vi "readCSV.vi"() -> ()   [LabVIEW 2020]
uses:
  <vilib>/Utility/file.llb/Read Delimited Spreadsheet (string).vi
panel:
  in  "Numeric 2":dbl
  out "Numeric":dbl
  out "String 3":string
  out "String 2":string
  out "Array":T1(array[cluster])
  in  "String":string
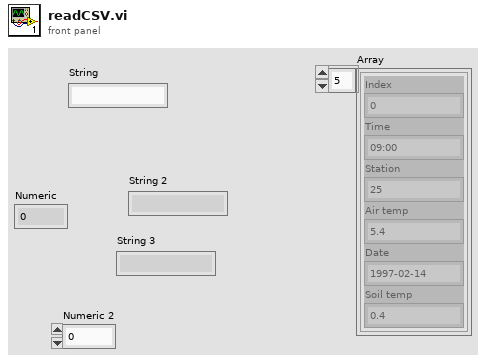
[diagram p1: front panel]
types:
  T1 = cluster{"Index":string, "Time":string, "Station":string, "Air temp":string, "Date":string, "Soil temp":string}[]
  T2 = cluster{"String 2":string, "String 3":string, "String 4":string, "String 5":string, "String 6":string, "String 7":string}
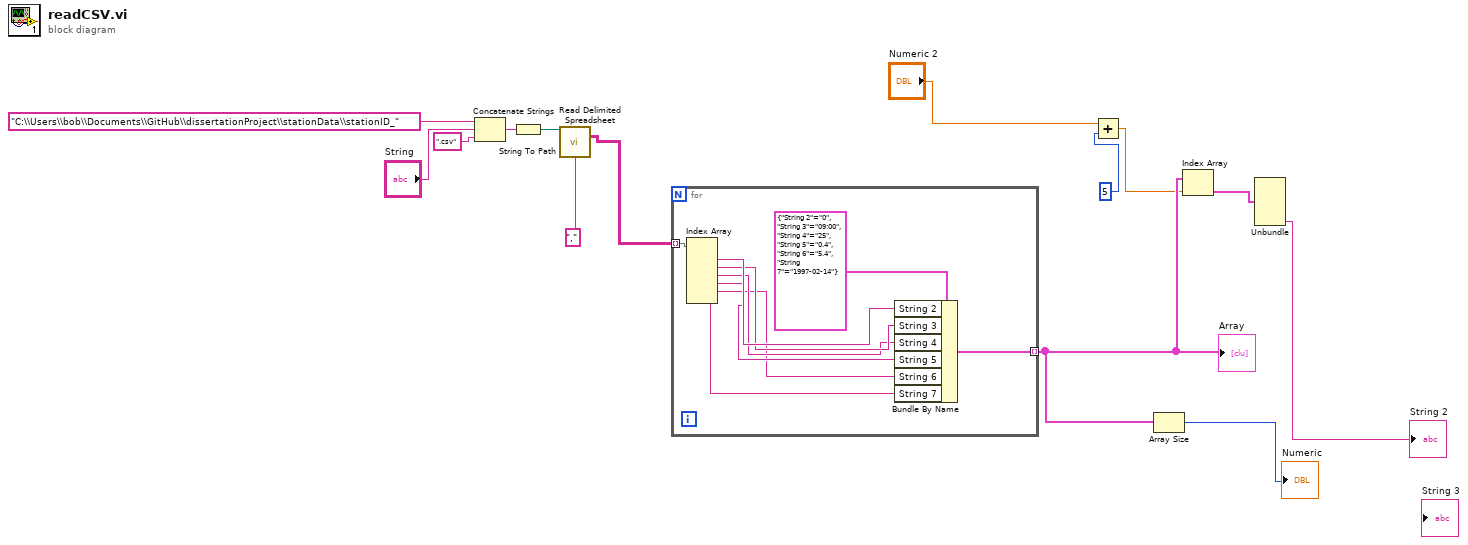
[diagram p0: block diagram]
diagram:
  n1 = Concatenate Strings("C:\\Users\\bob\\Documents\\GitHub\\dissertationProject\\stationData\\stationID_", "String", ".csv") -> (w11:string)
  n2 = String To Path(string=w11) -> (path=w10:path)
  n3 = call-poly <vilib>:"Read Delimited Spreadsheet.vi"("file path (dialog if empty)"=w10, "delimiter (\\t)"="," ("delimiter (\\t)")) -> ("all rows"=w8:string[][])  [unwired: 8 in, 5 out]
  n4 = for {
    tunnel: w8 -> [w23] mode=indexing
    tunnel: [w16] -> w6 mode=indexing
    n5 = Index Array(array=w23) -> (element #1=w21:string, element #2=w20:string, element #3=w19:string, element #4=w18:string, element #5=w17:string, element #6=w15:string)  [unwired: 6 in]
    n6 = Bundle By Name(cluster=T2 {"String 2"="0", "String 3"="09:00", "String 4"="25", "String 5"="0.4", "String 6"="5.4", "String 7"="1997-02-14"} ("Cluster"), "String 2"=w21, "String 3"=w20, "String 4"=w19, "String 5"=w18, "String 6"=w17, "String 7"=w15) -> (w16:T2)
  }
  "Array" <- w6
  n7 = Add(x="Numeric 2", y=5 ("index")) -> (x+y=w3:dbl)
  n8 = Array Size(array=w6) -> (size(s)=→"Numeric":i32)
  n9 = Index Array(array=w6, index=w3) -> (element=w5:T2)
  n10 = Unbundle(w5) -> ("String 7"=→"String 2":string)  [unwired: 5 out]
